vi "Wavefront Correction (SubVI).vi"(1 "Source Image Array":u8[](array[numeric]), 2 "Wavefront Correction":u8[](array[numeric])) -> (0 "Corrected Image Array":u8[](array[numeric]))   [LabVIEW 2010]
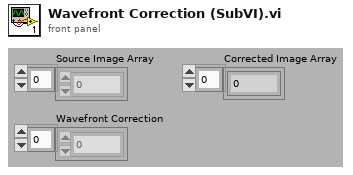
[diagram p1: front panel]
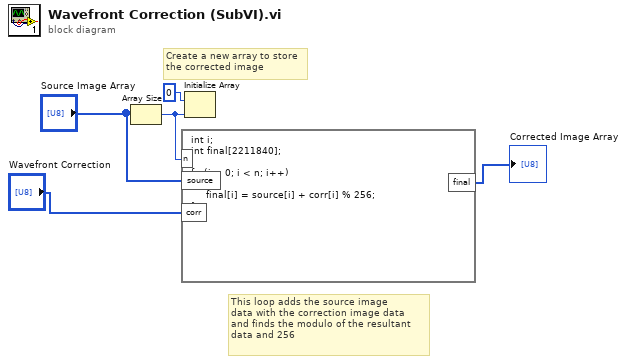
[diagram p0: block diagram]
diagram:
  # "This loop adds the source image\ndata with the correction image data\nand finds the modulo of the resultant\ndata and 256"
  # "Create a new array to store\nthe corrected image"
  n1 = Array Size(array="Source Image Array") -> (size(s)=w4:i32)
  n2 = formula code="int i;\nint final[2211840];\n\nfor(i = 0; i < n; i++)\n{\n     final[i] = source[i] + corr[i] % 256;\n}"("n"=w4, "source"="Source Image Array", "corr"="Wavefront Correction") -> ("final"=→"Corrected Image Array":i32[])
  n3 = Initialize Array(u8 0, w4) -> ()  [unwired: 1 out]
